vi "Decript UDP Message.vi"(8 "Error In":errorcluster, 10 "UDP Message":u8[](array[numeric])) -> (0 "Error Out":errorcluster, 2 "Analog Input":dbl[](array[numeric]), 3 "Digital Input":bool[](array[boolean]))   [LabVIEW 2019, in "HMI.lvlib"]
uses:
  HMI.lvlib
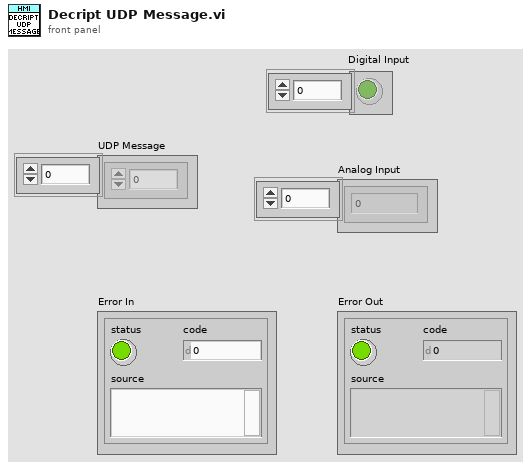
[diagram p1: front panel]
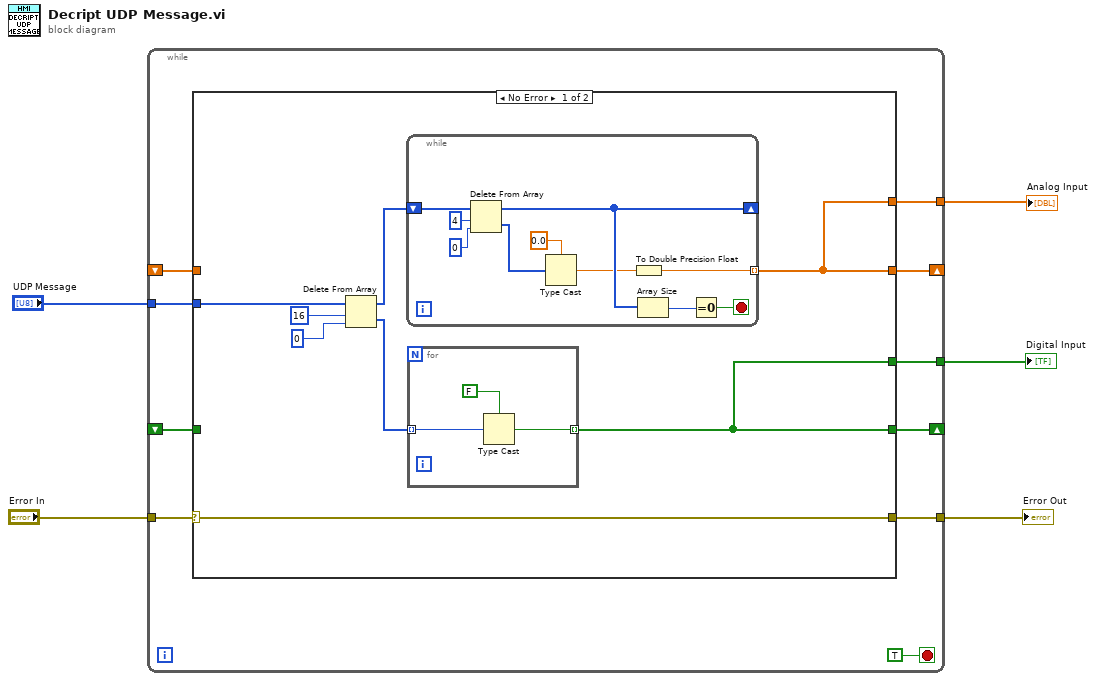
[diagram p0: block diagram]
diagram:
  n1 = while {
    tunnel: "UDP Message" -> [w15]
    tunnel: [w14] -> w4
    tunnel: [w13] -> w3
    tunnel: "Error In" -> [w11]
    tunnel: [w10] -> w1
    shift-right: [w9] -> _
    shift-left: _ -> [w8]
    shift-right: [w7] -> _
    shift-left: _ -> [w6]
    stop <- TRUE stop-if-true
    n2 = case shown="No Error" w11 {
      selector: w11 -> [w18 w37]
      tunnel: w15 -> [w21 _]
      tunnel: [w17 w38] -> w14
      tunnel: [w16 w39] -> w13
      tunnel: [w18 w37] -> w10
      tunnel: [w17 w38] -> w9
      tunnel: w8 -> [_ w38]
      tunnel: [w16 w39] -> w7
      tunnel: w6 -> [_ w39]
      frame No Error {
        n3 = Delete From Array(array=w21, length=16, index=0) -> (deleted portion=w20:u8[], array with subset deleted=w19:u8[])
        n4 = while {
          shift-right: [w26] -> _
          shift-left: w19 -> [w33]
          tunnel: [w24] -> w16 mode=indexing
          stop <- w28 stop-if-true
          n5 = Delete From Array(array=w33, length=4, index=0) -> (deleted portion=w30:u8[], array with subset deleted=w26:u8[])
          n6 = Type Cast(type=sgl 0.0, x=w30) -> (*(type *) &x=w25:sgl)
          n7 = To Double Precision Float(number=w25) -> (double precision float=w24:dbl)
          n8 = Array Size(array=w26) -> (size(s)=w27:i32)
          n9 = Equal To 0?(x=w27) -> (x = 0?=w28:bool)
        }
        n10 = for {
          tunnel: w20 -> [w36] mode=indexing
          tunnel: [w34] -> w17 mode=indexing
          n11 = Type Cast(type=FALSE, x=w36) -> (*(type *) &x=w34:bool)
        }
      }
      frame Error {
      }
    }
  }
  "Error Out" <- w1
  "Digital Input" <- w4
  "Analog Input" <- w3
